vi "BRig_RT__Case_Exp__State_initTrial__LC_ENL__v4.vi"(6 "input_arrTrig":bool[](array[boolean]), 8 "input_dataTrial":u16[][](array[numeric]), 9 "input_dataExp":u16[](array[numeric]), 10 "input_dataLC":u16[](array[numeric]), 11 "input_dataCurrent":u16[](array[numeric])) -> (0 "output_dataTrial":u16[][](array[numeric]), 3 "output_dataCurrent":u16[](array[numeric]), 4 "output_arrTrig":bool[](array[boolean]))   [LabVIEW 2014]
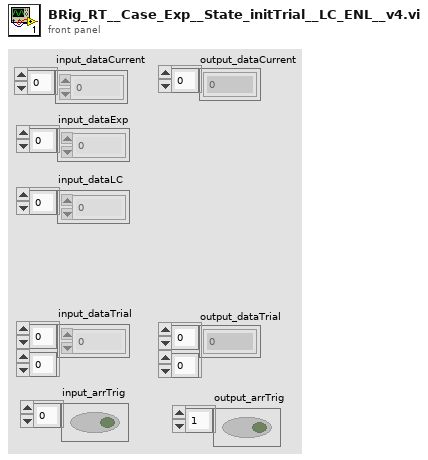
[diagram p1: front panel]
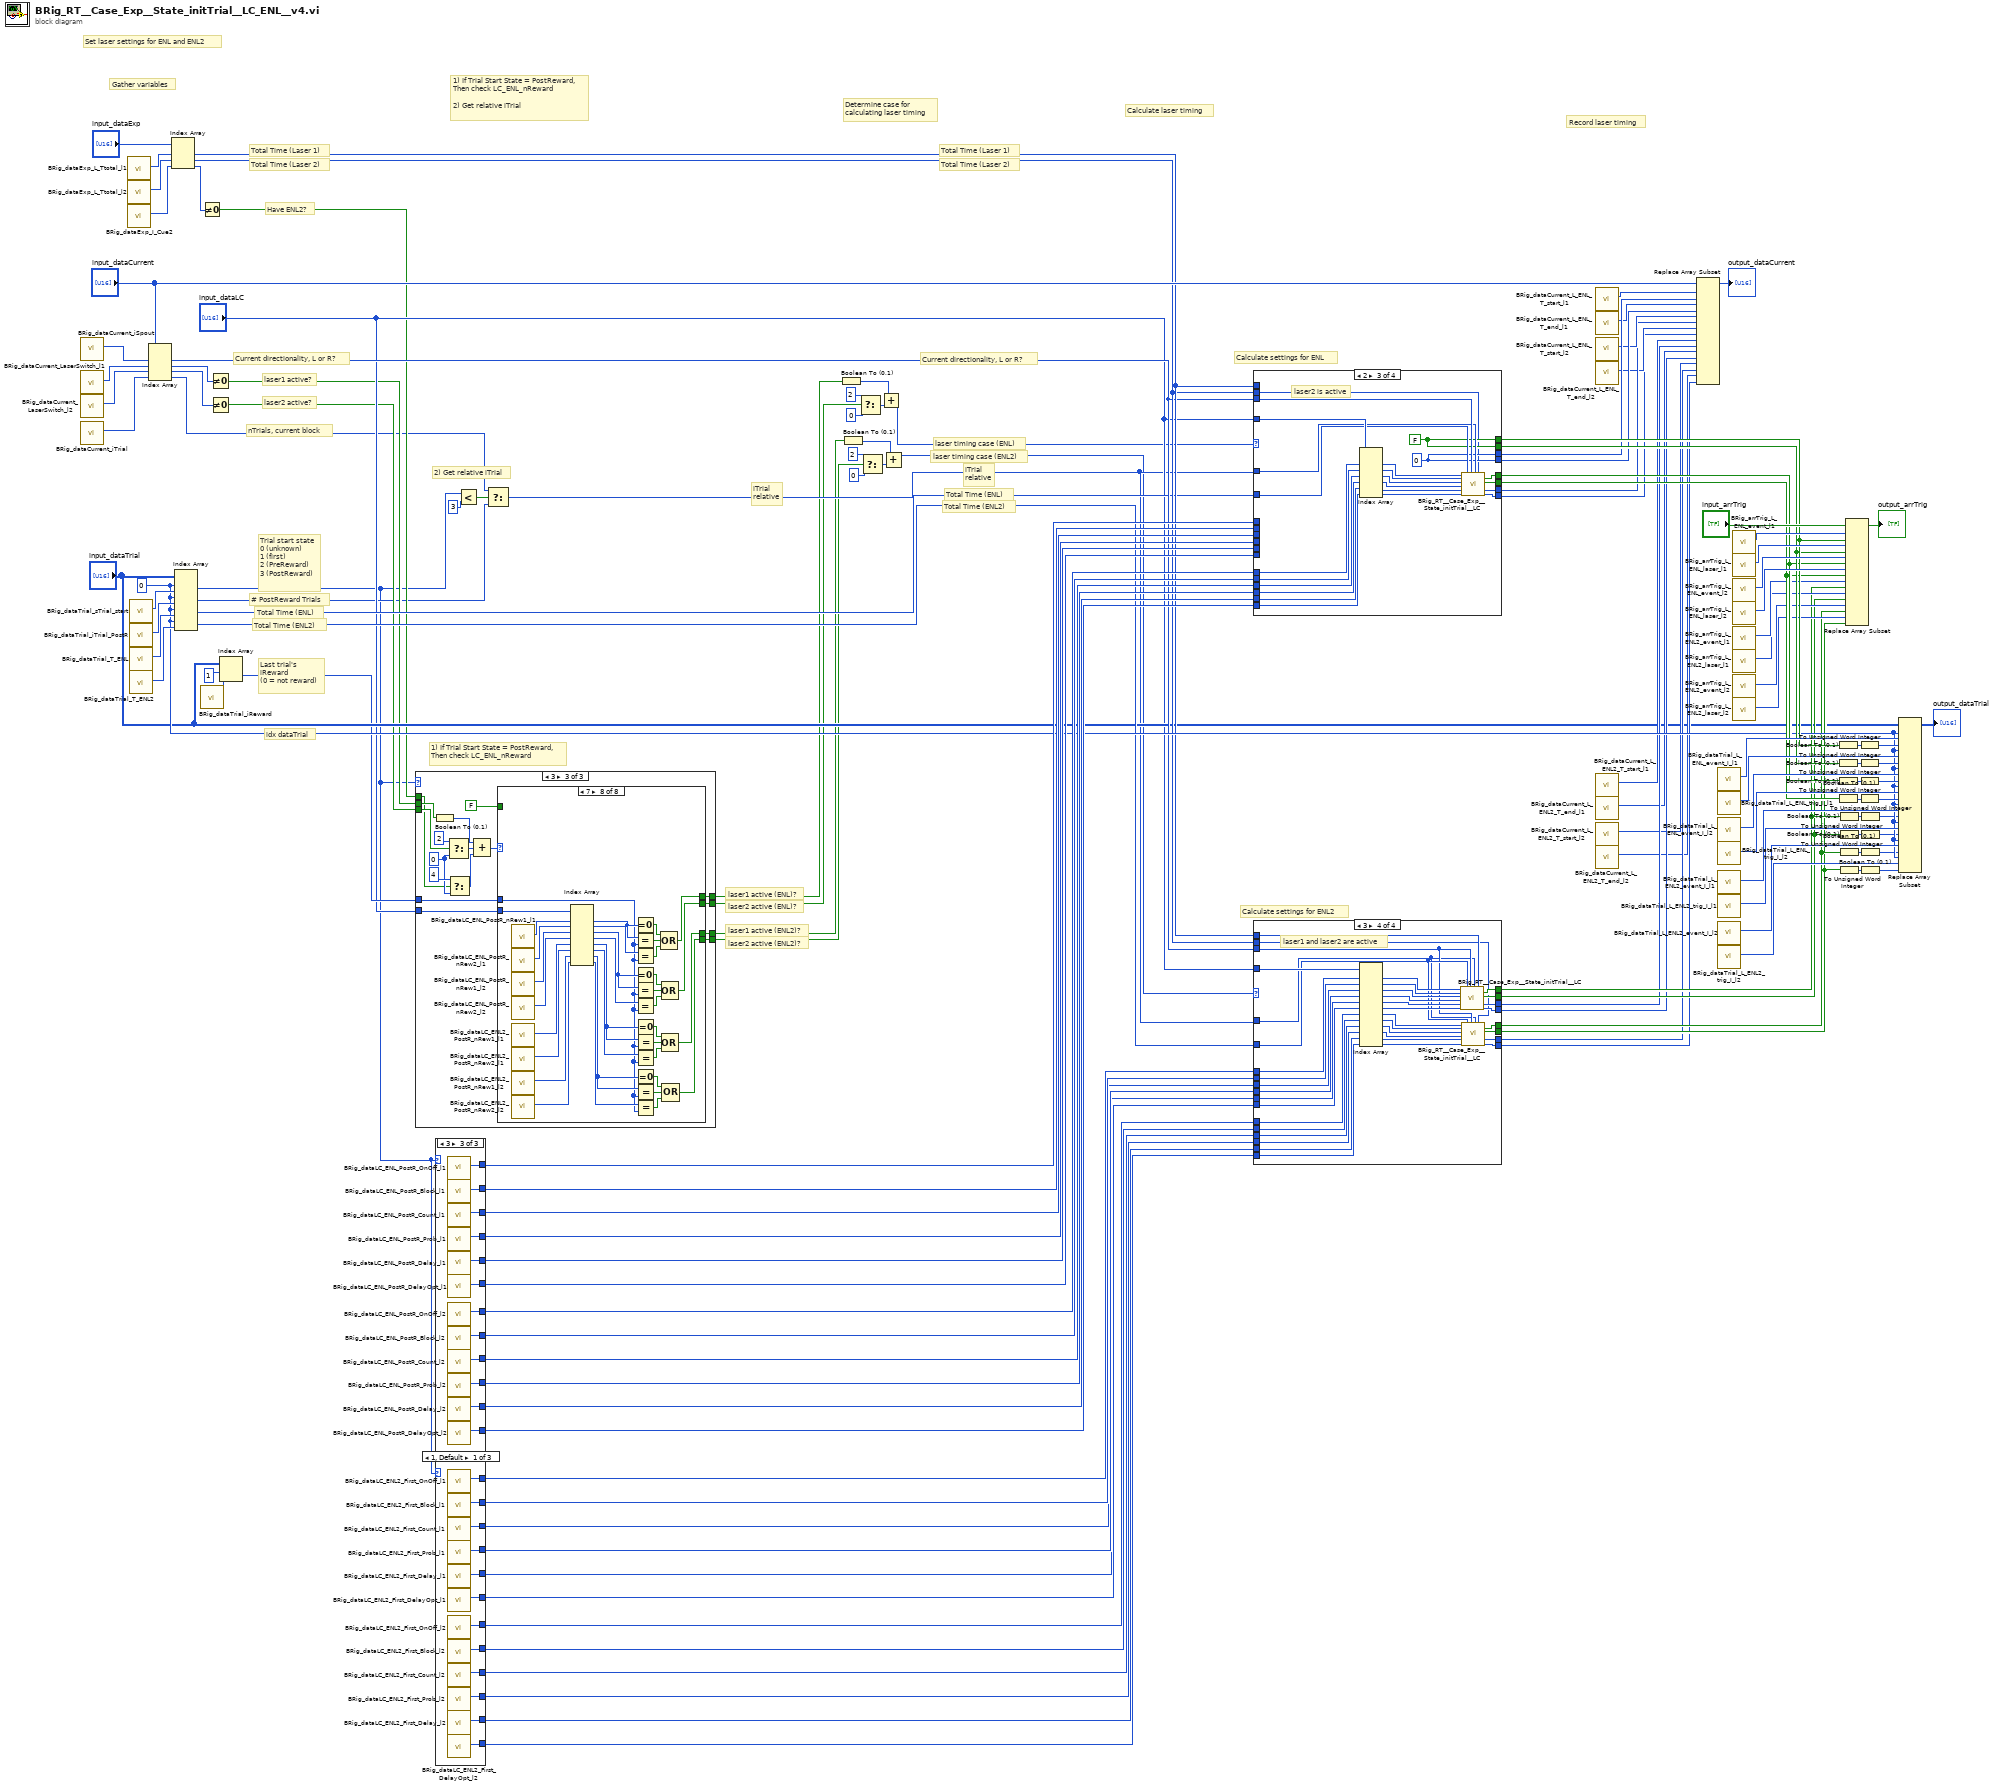
[diagram p0: block diagram]
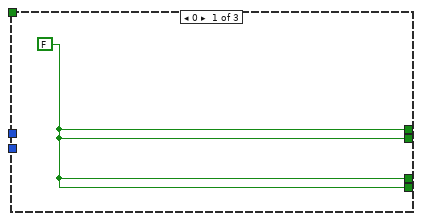
[diagram p2: hidden frame]
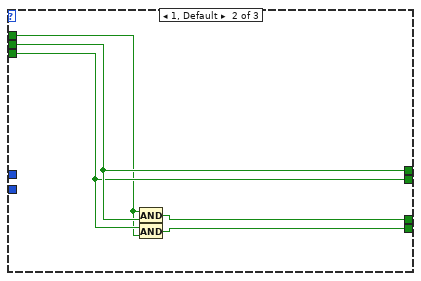
[diagram p3: hidden frame]
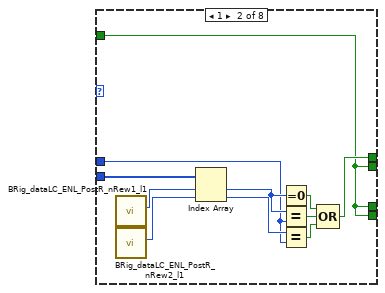
[diagram p5: hidden frame]
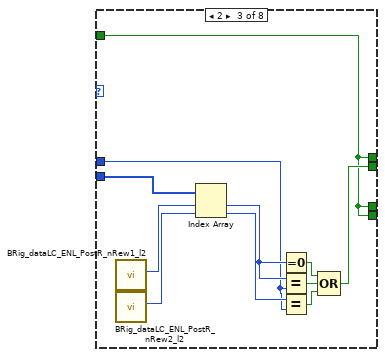
[diagram p6: hidden frame]
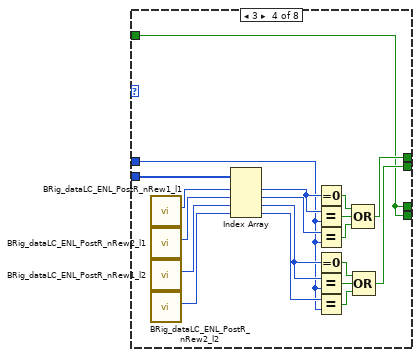
[diagram p7: hidden frame]
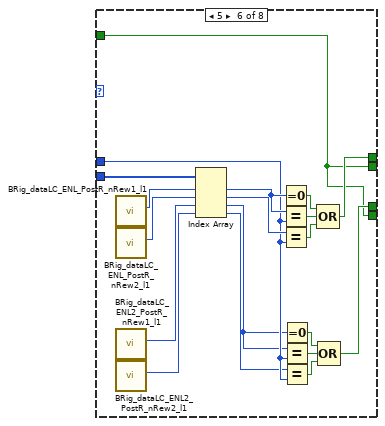
[diagram p9: hidden frame]
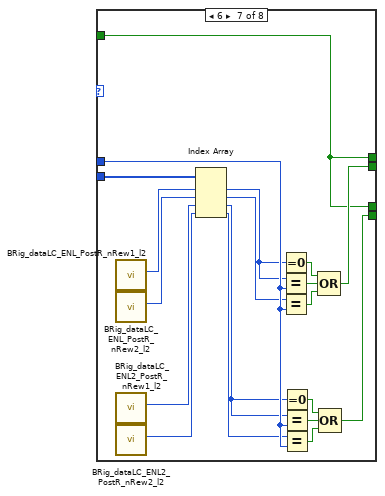
[diagram p10: hidden frame]
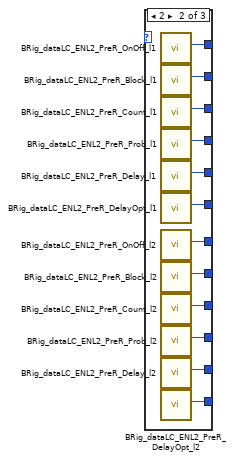
[diagram p11: hidden frame]
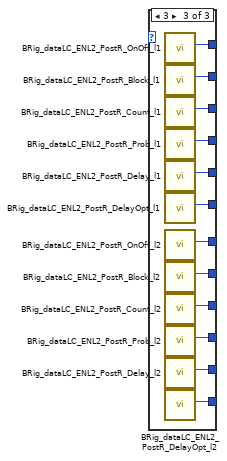
[diagram p12: hidden frame]
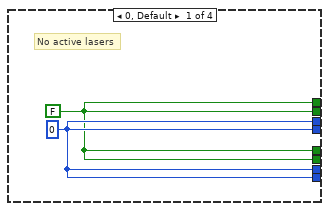
[diagram p13: hidden frame]
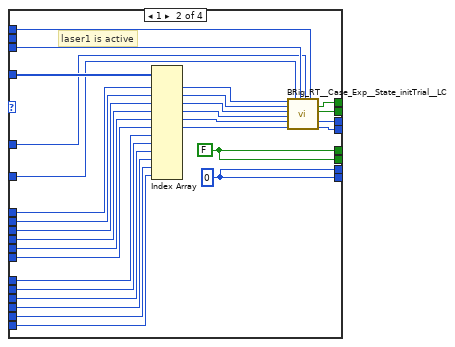
[diagram p14: hidden frame]
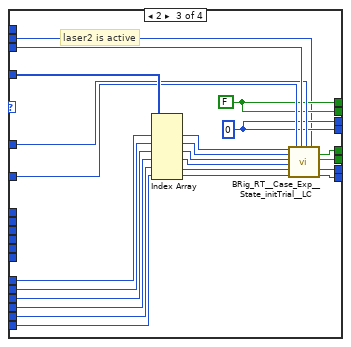
[diagram p15: hidden frame]
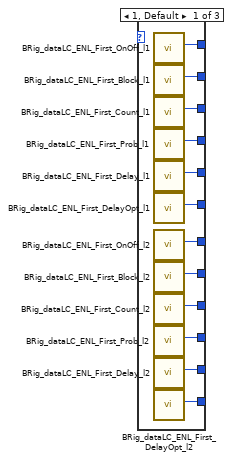
[diagram p16: hidden frame]
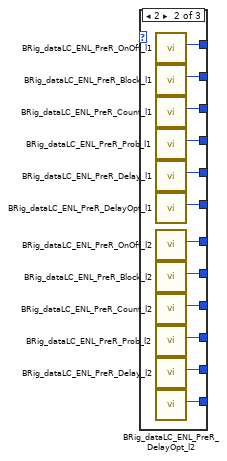
[diagram p17: hidden frame]
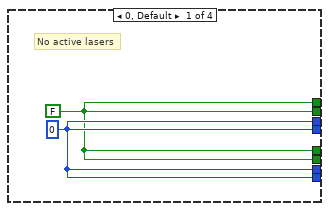
[diagram p18: hidden frame]
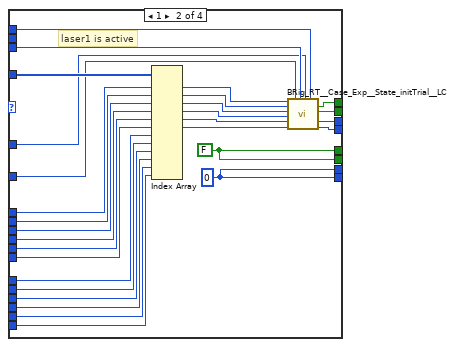
[diagram p19: hidden frame]
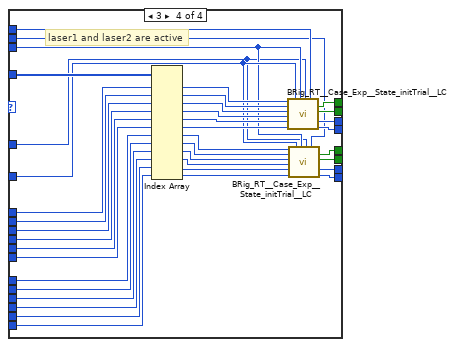
[diagram p20: hidden frame]
diagram:
  w61 = 0
  # "Record laser timing"
  # "Calculate laser timing"
  # "Total Time (ENL2)"
  # "Total Time (ENL)"
  # "iTrial\nrelative"
  # "Total Time (Laser 2)"
  # "Total Time (Laser 1)"
  # "Current directionality, L or R?"
  # "laser timing case (ENL2)"
  # "Determine case for\ncalculating laser timing"
  # "2) Get relative iTrial"
  # "1) If Trial Start State = PostReward,\nThen check LC_ENL_nReward"
  # "laser2 active (ENL2)?"
  # "laser1 active (ENL2)?"
  # "laser2 active (ENL)?"
  # "laser1 active (ENL)?"
  # "1) If Trial Start State = PostReward,\nThen check LC_ENL_nReward\n\n2) Get relative iTrial"
  # "Gather variables"
  # "Last trial's\niReward\n(0 = not reward)"
  # "nTrials, current block"
  # "idx dataTrial"
  # "Total Time (ENL2)"
  # "Total Time (ENL)"
  # "# PostReward Trials"
  # "Current directionality, L or R?"
  # "Have ENL2?"
  # "Total Time (Laser 2)"
  # "Total Time (Laser 1)"
  # "Calculate settings for ENL2"
  # "Calculate settings for ENL"
  # "Set laser settings for ENL and ENL2"
  # "iTrial\nrelative"
  # "laser timing case (ENL)"
  # "Trial start state\n0 (unknown)\n1 (first)\n2 (PreReward)\n3 (PostReward)"
  # "laser2 active?"
  # "laser1 active?"
  n1 = call "BRig_dataCurrent_iSpout.vi"() -> ("output_iSpout"=w125:i32)  [unwired: 11 in]
  n2 = call "BRig_dataCurrent_LaserSwitch_l1.vi"() -> ("output_LaserSwitch_l1"=w134:i32)  [unwired: 11 in]
  n3 = call "BRig_dataCurrent_LaserSwitch_l2.vi"() -> ("output_LaserSwitch_l2"=w133:i32)  [unwired: 11 in]
  n4 = call "BRig_dataCurrent_iTrial.vi"() -> ("output_iTrial"=w74:i32)  [unwired: 11 in]
  n5 = call "BRig_dataExp_L_Ttotal_l1.vi"() -> ("output_L_Ttotal_l1"=w78:i32)  [unwired: 11 in]
  n6 = call "BRig_dataExp_L_Ttotal_l2.vi"() -> ("output_L_Ttotal_l2"=w79:i32)  [unwired: 11 in]
  n7 = call "BRig_dataExp_I_Cue2.vi"() -> ("output_I_Cue2"=w28:i32)  [unwired: 11 in]
  n8 = call "BRig_dataTrial_sTrial_start.vi"() -> ("output_sTrial_start"=w130:i32)  [unwired: 11 in]
  n9 = call "BRig_dataTrial_iTrial_PostR.vi"() -> ("output_iTrial_PostR"=w75:i32)  [unwired: 11 in]
  n10 = call "BRig_dataTrial_T_ENL.vi"() -> ("output_T_ENL"=w76:i32)  [unwired: 11 in]
  n11 = call "BRig_dataTrial_T_ENL2.vi"() -> ("output_T_ENL2"=w73:i32)  [unwired: 11 in]
  n12 = Index Array(array="input_dataCurrent", index #1=w125, index #2=w134, index #3=w133, index #4=w74) -> (element #1=w53:u16, element #2=w132:u16, element #3=w131:u16, element #4=w14:u16)
  n13 = Index Array(array="input_dataExp", index #1=w78, index #2=w79, index #3=w28) -> (element #1=w55:u16, element #2=w54:u16, element #3=w27:u16)
  n14 = Index Array(array="input_dataTrial", index (row) #1=w61, index (col) #1=w130, index (row) #2=w61, index (col) #2=w75, index (row) #3=w61, index (col) #3=w76, index (row) #4=w61, index (col) #4=w73) -> (element #1=w12:u16, element #2=w13:u16, element #3=w26:u16, element #4=w25:u16)
  n15 = Not Equal To 0?(x=w27) -> (x != 0?=w17:bool)
  n16 = call "BRig_dataTrial_iReward.vi"() -> ("output_iReward"=w23:i32)  [unwired: 11 in]
  n17 = Not Equal To 0?(x=w132) -> (x != 0?=w18:bool)
  n18 = Not Equal To 0?(x=w131) -> (x != 0?=w19:bool)
  n19 = Index Array(array="input_dataTrial", index (row)=1 ("disabled index (row)"), index (col)=w23) -> (element=w21:u16)
  n20 = case shown="3" w12 {
    tunnel: w21 -> [_ _ w149]
    tunnel: "input_dataLC" -> [_ _ w150]
    tunnel: w19 -> [_ w139 w142]
    tunnel: w18 -> [_ w140 w143]
    tunnel: w17 -> [_ w138 w141]
    tunnel: [w135 w140 w148] -> w10
    tunnel: [w135 w139 w147] -> w9
    tunnel: [w135 w137 w146] -> w4
    tunnel: [w135 w136 w145] -> w3
    frame 0 {
      w135 = FALSE
    }
    frame 1, Default {
      n21 = And(x=w138, y=w140) -> (x .and. y?=w137:bool)
      n22 = And(x=w139, y=w138) -> (x .and. y?=w136:bool)
    }
    frame 3 {
      w155 = i16 0 ("f")
      n23 = Boolean To (0,1)(Boolean=w143) -> (0, 1=w153:i16)
      n24 = Select(t=i16 2, s=w142, f=w155) -> (s? t:f=w154:i16)
      n25 = Select(t=i16 4, s=w141, f=w155) -> (s? t:f=w152:i16)
      n26 = Compound Arithmetic op=ADD(w153, w154, w152) -> (w151:i16)
      n27 = case shown="7" w151 {
        tunnel: w150 -> [_ w162 w173 w185 _ w212 w235 w258]
        tunnel: w149 -> [_ w161 w172 w184 _ w208 w231 w243]
        tunnel: [w158 w160 w170 w183 w200 w207 w228 w242] -> w148
        tunnel: [w158 w159 w171 w182 w200 w205 w230 w241] -> w147
        tunnel: [w158 w159 w170 w181 w200 w206 w228 w240] -> w146
        tunnel: [w158 w159 w170 w181 w200 w205 w229 w239] -> w145
        tunnel: FALSE -> [w158 w159 w170 w181 w200 w205 w228 _]
        frame 0, Default {
        }
        frame 1 {
          n28 = call "BRig_dataLC_ENL_PostR_nRew1_l1.vi"() -> ("output_ENL_PostR_nRew1_l1"=w169:i32)  [unwired: 11 in]
          n29 = call "BRig_dataLC_ENL_PostR_nRew2_l1.vi"() -> ("output_ENL_PostR_nRew2_l1"=w168:i32)  [unwired: 11 in]
          n30 = Index Array(array=w162, index #1=w169, index #2=w168) -> (element #1=w164:u16, element #2=w163:u16)
          n31 = Equal To 0?(x=w164) -> (x = 0?=w165:bool)
          n32 = Equal?(x=w164, y=w161) -> (x = y?=w166:bool)
          n33 = Equal?(x=w163, y=w161) -> (x = y?=w167:bool)
          n34 = Compound Arithmetic op=OR(w165, w166, w167) -> (w160:bool)
        }
        frame 2 {
          n35 = call "BRig_dataLC_ENL_PostR_nRew1_l2.vi"() -> ("output_ENL_PostR_nRew1_l2"=w180:i32)  [unwired: 11 in]
          n36 = call "BRig_dataLC_ENL_PostR_nRew2_l2.vi"() -> ("output_ENL_PostR_nRew2_l2"=w179:i32)  [unwired: 11 in]
          n37 = Index Array(array=w173, index #1=w180, index #2=w179) -> (element #1=w174:u16, element #2=w175:u16)
          n38 = Equal To 0?(x=w174) -> (x = 0?=w177:bool)
          n39 = Equal?(x=w174, y=w172) -> (x = y?=w176:bool)
          n40 = Equal?(x=w175, y=w172) -> (x = y?=w178:bool)
          n41 = Compound Arithmetic op=OR(w177, w176, w178) -> (w171:bool)
        }
        frame 3 {
          n42 = call "BRig_dataLC_ENL_PostR_nRew1_l1.vi"() -> ("output_ENL_PostR_nRew1_l1"=w199:i32)  [unwired: 11 in]
          n43 = call "BRig_dataLC_ENL_PostR_nRew2_l1.vi"() -> ("output_ENL_PostR_nRew2_l1"=w198:i32)  [unwired: 11 in]
          n44 = call "BRig_dataLC_ENL_PostR_nRew1_l2.vi"() -> ("output_ENL_PostR_nRew1_l2"=w197:i32)  [unwired: 11 in]
          n45 = call "BRig_dataLC_ENL_PostR_nRew2_l2.vi"() -> ("output_ENL_PostR_nRew2_l2"=w196:i32)  [unwired: 11 in]
          n46 = Index Array(array=w185, index #1=w199, index #2=w198, index #3=w197, index #4=w196) -> (element #1=w189:u16, element #2=w188:u16, element #3=w186:u16, element #4=w187:u16)
          n47 = Equal To 0?(x=w189) -> (x = 0?=w190:bool)
          n48 = Equal?(x=w189, y=w184) -> (x = y?=w191:bool)
          n49 = Equal?(x=w188, y=w184) -> (x = y?=w192:bool)
          n50 = Equal To 0?(x=w186) -> (x = 0?=w194:bool)
          n51 = Equal?(x=w186, y=w184) -> (x = y?=w193:bool)
          n52 = Equal?(x=w187, y=w184) -> (x = y?=w195:bool)
          n53 = Compound Arithmetic op=OR(w190, w191, w192) -> (w183:bool)
          n54 = Compound Arithmetic op=OR(w194, w193, w195) -> (w182:bool)
        }
        frame 4 {
        }
        frame 5 {
          n55 = call "BRig_dataLC_ENL_PostR_nRew1_l1.vi"() -> ("output_ENL_PostR_nRew1_l1"=w219:i32)  [unwired: 11 in]
          n56 = call "BRig_dataLC_ENL_PostR_nRew2_l1.vi"() -> ("output_ENL_PostR_nRew2_l1"=w218:i32)  [unwired: 11 in]
          n57 = call "BRig_dataLC_ENL2_PostR_nRew1_l1.vi"() -> ("output_ENL2_PostR_nRew1_l1"=w204:i32)  [unwired: 11 in]
          n58 = call "BRig_dataLC_ENL2_PostR_nRew2_l1.vi"() -> ("output_ENL2_PostR_nRew2_l1"=w203:i32)  [unwired: 11 in]
          n59 = Index Array(array=w212, index #1=w219, index #2=w218, index #3=w204, index #4=w203) -> (element #1=w214:u16, element #2=w213:u16, element #3=w202:u16, element #4=w201:u16)
          n60 = Equal To 0?(x=w214) -> (x = 0?=w215:bool)
          n61 = Equal?(x=w214, y=w208) -> (x = y?=w216:bool)
          n62 = Equal?(x=w213, y=w208) -> (x = y?=w217:bool)
          n63 = Equal To 0?(x=w202) -> (x = 0?=w211:bool)
          n64 = Equal?(x=w202, y=w208) -> (x = y?=w210:bool)
          n65 = Equal?(x=w201, y=w208) -> (x = y?=w209:bool)
          n66 = Compound Arithmetic op=OR(w215, w216, w217) -> (w207:bool)
          n67 = Compound Arithmetic op=OR(w211, w210, w209) -> (w206:bool)
        }
        frame 6 {
          n68 = call "BRig_dataLC_ENL_PostR_nRew1_l2.vi"() -> ("output_ENL_PostR_nRew1_l2"=w227:i32)  [unwired: 11 in]
          n69 = call "BRig_dataLC_ENL_PostR_nRew2_l2.vi"() -> ("output_ENL_PostR_nRew2_l2"=w226:i32)  [unwired: 11 in]
          n70 = call "BRig_dataLC_ENL2_PostR_nRew1_l2.vi"() -> ("output_ENL2_PostR_nRew1_l2"=w223:i32)  [unwired: 11 in]
          n71 = call "BRig_dataLC_ENL2_PostR_nRew2_l2.vi"() -> ("output_ENL2_PostR_nRew2_l2"=w222:i32)  [unwired: 11 in]
          n72 = Index Array(array=w235, index #1=w227, index #2=w226, index #3=w223, index #4=w222) -> (element #1=w225:u16, element #2=w224:u16, element #3=w221:u16, element #4=w220:u16)
          n73 = Equal To 0?(x=w225) -> (x = 0?=w237:bool)
          n74 = Equal?(x=w225, y=w231) -> (x = y?=w236:bool)
          n75 = Equal?(x=w224, y=w231) -> (x = y?=w238:bool)
          n76 = Equal To 0?(x=w221) -> (x = 0?=w233:bool)
          n77 = Equal?(x=w221, y=w231) -> (x = y?=w234:bool)
          n78 = Equal?(x=w220, y=w231) -> (x = y?=w232:bool)
          n79 = Compound Arithmetic op=OR(w237, w236, w238) -> (w230:bool)
          n80 = Compound Arithmetic op=OR(w233, w234, w232) -> (w229:bool)
        }
        frame 7 {
          n81 = call "BRig_dataLC_ENL_PostR_nRew1_l1.vi"() -> ("output_ENL_PostR_nRew1_l1"=w272:i32)  [unwired: 11 in]
          n82 = call "BRig_dataLC_ENL_PostR_nRew2_l1.vi"() -> ("output_ENL_PostR_nRew2_l1"=w271:i32)  [unwired: 11 in]
          n83 = call "BRig_dataLC_ENL_PostR_nRew1_l2.vi"() -> ("output_ENL_PostR_nRew1_l2"=w270:i32)  [unwired: 11 in]
          n84 = call "BRig_dataLC_ENL_PostR_nRew2_l2.vi"() -> ("output_ENL_PostR_nRew2_l2"=w269:i32)  [unwired: 11 in]
          n85 = call "BRig_dataLC_ENL2_PostR_nRew1_l1.vi"() -> ("output_ENL2_PostR_nRew1_l1"=w257:i32)  [unwired: 11 in]
          n86 = call "BRig_dataLC_ENL2_PostR_nRew2_l1.vi"() -> ("output_ENL2_PostR_nRew2_l1"=w256:i32)  [unwired: 11 in]
          n87 = call "BRig_dataLC_ENL2_PostR_nRew1_l2.vi"() -> ("output_ENL2_PostR_nRew1_l2"=w255:i32)  [unwired: 11 in]
          n88 = call "BRig_dataLC_ENL2_PostR_nRew2_l2.vi"() -> ("output_ENL2_PostR_nRew2_l2"=w254:i32)  [unwired: 11 in]
          n89 = Index Array(array=w258, index #1=w272, index #2=w271, index #3=w270, index #4=w269, index #5=w257, index #6=w256, index #7=w255, index #8=w254) -> (element #1=w262:u16, element #2=w261:u16, element #3=w259:u16, element #4=w260:u16, element #5=w247:u16, element #6=w246:u16, element #7=w244:u16, element #8=w245:u16)
          n90 = Equal To 0?(x=w262) -> (x = 0?=w263:bool)
          n91 = Equal?(x=w262, y=w243) -> (x = y?=w264:bool)
          n92 = Equal?(x=w261, y=w243) -> (x = y?=w265:bool)
          n93 = Equal To 0?(x=w259) -> (x = 0?=w267:bool)
          n94 = Equal?(x=w259, y=w243) -> (x = y?=w266:bool)
          n95 = Equal?(x=w260, y=w243) -> (x = y?=w268:bool)
          n96 = Equal To 0?(x=w247) -> (x = 0?=w253:bool)
          n97 = Equal?(x=w247, y=w243) -> (x = y?=w252:bool)
          n98 = Equal?(x=w246, y=w243) -> (x = y?=w251:bool)
          n99 = Equal To 0?(x=w244) -> (x = 0?=w249:bool)
          n100 = Equal?(x=w244, y=w243) -> (x = y?=w250:bool)
          n101 = Equal?(x=w245, y=w243) -> (x = y?=w248:bool)
          n102 = Compound Arithmetic op=OR(w263, w264, w265) -> (w242:bool)
          n103 = Compound Arithmetic op=OR(w267, w266, w268) -> (w241:bool)
          n104 = Compound Arithmetic op=OR(w253, w252, w251) -> (w240:bool)
          n105 = Compound Arithmetic op=OR(w249, w250, w248) -> (w239:bool)
        }
      }
    }
  }
  n106 = case shown="3" w12 {
    tunnel: [w284 w296 w308] -> w91
    tunnel: [w283 w295 w297] -> w90
    tunnel: [w282 w294 w298] -> w89
    tunnel: [w281 w293 w299] -> w88
    tunnel: [w280 w292 w300] -> w87
    tunnel: [w279 w291 w301] -> w86
    tunnel: [w278 w290 w307] -> w85
    tunnel: [w277 w289 w306] -> w84
    tunnel: [w276 w288 w305] -> w83
    tunnel: [w275 w287 w304] -> w82
    tunnel: [w274 w286 w303] -> w81
    tunnel: [w273 w285 w302] -> w80
    frame 1, Default {
      n107 = call "BRig_dataLC_ENL_First_OnOff_l1.vi"() -> ("output_ENL_First_OnOff"=w284:i32)  [unwired: 11 in]
      n108 = call "BRig_dataLC_ENL_First_Block_l1.vi"() -> ("output_ENL_First_Block"=w283:i32)  [unwired: 11 in]
      n109 = call "BRig_dataLC_ENL_First_Count_l1.vi"() -> ("output_ENL_First_Count"=w282:i32)  [unwired: 11 in]
      n110 = call "BRig_dataLC_ENL_First_Prob_l1.vi"() -> ("output_ENL_First_Prob"=w281:i32)  [unwired: 11 in]
      n111 = call "BRig_dataLC_ENL_First_Delay_l1.vi"() -> ("output_ENL_First_Delay"=w280:i32)  [unwired: 11 in]
      n112 = call "BRig_dataLC_ENL_First_DelayOpt_l1.vi"() -> ("output_ENL_First_DelayOpt"=w279:i32)  [unwired: 11 in]
      n113 = call "BRig_dataLC_ENL_First_OnOff_l2.vi"() -> ("output_ENL_First_OnOff_l2"=w278:i32)  [unwired: 11 in]
      n114 = call "BRig_dataLC_ENL_First_Block_l2.vi"() -> ("output_ENL_First_Block_l2"=w277:i32)  [unwired: 11 in]
      n115 = call "BRig_dataLC_ENL_First_Count_l2.vi"() -> ("output_ENL_First_Count_l2"=w276:i32)  [unwired: 11 in]
      n116 = call "BRig_dataLC_ENL_First_Prob_l2.vi"() -> ("output_ENL_First_Prob_l2"=w275:i32)  [unwired: 11 in]
      n117 = call "BRig_dataLC_ENL_First_Delay_l2.vi"() -> ("output_ENL_First_Delay_l2"=w274:i32)  [unwired: 11 in]
      n118 = call "BRig_dataLC_ENL_First_DelayOpt_l2.vi"() -> ("output_ENL_First_DelayOpt_l2"=w273:i32)  [unwired: 11 in]
    }
    frame 2 {
      n119 = call "BRig_dataLC_ENL_PreR_OnOff_l1.vi"() -> ("output_ENL_PreR_OnOff"=w296:i32)  [unwired: 11 in]
      n120 = call "BRig_dataLC_ENL_PreR_Block_l1.vi"() -> ("output_ENL_PreR_Block"=w295:i32)  [unwired: 11 in]
      n121 = call "BRig_dataLC_ENL_PreR_Count_l1.vi"() -> ("output_ENL_PreR_Count"=w294:i32)  [unwired: 11 in]
      n122 = call "BRig_dataLC_ENL_PreR_Prob_l1.vi"() -> ("output_ENL_PreR_Prob"=w293:i32)  [unwired: 11 in]
      n123 = call "BRig_dataLC_ENL_PreR_Delay_l1.vi"() -> ("output_ENL_PreR_Delay"=w292:i32)  [unwired: 11 in]
      n124 = call "BRig_dataLC_ENL_PreR_DelayOpt_l1.vi"() -> ("output_ENL_PreR_DelayOpt"=w291:i32)  [unwired: 11 in]
      n125 = call "BRig_dataLC_ENL_PreR_OnOff_l2.vi"() -> ("output_ENL_PreR_OnOff_l2"=w290:i32)  [unwired: 11 in]
      n126 = call "BRig_dataLC_ENL_PreR_Block_l2.vi"() -> ("output_ENL_PreR_Block_l2"=w289:i32)  [unwired: 11 in]
      n127 = call "BRig_dataLC_ENL_PreR_Count_l2.vi"() -> ("output_ENL_PreR_Count_l2"=w288:i32)  [unwired: 11 in]
      n128 = call "BRig_dataLC_ENL_PreR_Prob_l2.vi"() -> ("output_ENL_PreR_Prob_l2"=w287:i32)  [unwired: 11 in]
      n129 = call "BRig_dataLC_ENL_PreR_Delay_l2.vi"() -> ("output_ENL_PreR_Delay_l2"=w286:i32)  [unwired: 11 in]
      n130 = call "BRig_dataLC_ENL_PreR_DelayOpt_l2.vi"() -> ("output_ENL_PreR_DelayOpt_l2"=w285:i32)  [unwired: 11 in]
    }
    frame 3 {
      n131 = call "BRig_dataLC_ENL_PostR_OnOff_l1.vi"() -> ("output_ENL_PostR_OnOff"=w308:i32)  [unwired: 11 in]
      n132 = call "BRig_dataLC_ENL_PostR_Block_l1.vi"() -> ("output_ENL_PostR_Block"=w297:i32)  [unwired: 11 in]
      n133 = call "BRig_dataLC_ENL_PostR_Count_l1.vi"() -> ("output_ENL_PostR_Count"=w298:i32)  [unwired: 11 in]
      n134 = call "BRig_dataLC_ENL_PostR_Prob_l1.vi"() -> ("output_ENL_PostR_Prob"=w299:i32)  [unwired: 11 in]
      n135 = call "BRig_dataLC_ENL_PostR_Delay_l1.vi"() -> ("output_ENL_PostR_Delay"=w300:i32)  [unwired: 11 in]
      n136 = call "BRig_dataLC_ENL_PostR_DelayOpt_l1.vi"() -> ("output_ENL_PostR_DelayOpt"=w301:i32)  [unwired: 11 in]
      n137 = call "BRig_dataLC_ENL_PostR_OnOff_l2.vi"() -> ("output_ENL_PostR_OnOff_l2"=w307:i32)  [unwired: 11 in]
      n138 = call "BRig_dataLC_ENL_PostR_Block_l2.vi"() -> ("output_ENL_PostR_Block_l2"=w306:i32)  [unwired: 11 in]
      n139 = call "BRig_dataLC_ENL_PostR_Count_l2.vi"() -> ("output_ENL_PostR_Count_l2"=w305:i32)  [unwired: 11 in]
      n140 = call "BRig_dataLC_ENL_PostR_Prob_l2.vi"() -> ("output_ENL_PostR_Prob_l2"=w304:i32)  [unwired: 11 in]
      n141 = call "BRig_dataLC_ENL_PostR_Delay_l2.vi"() -> ("output_ENL_PostR_Delay_l2"=w303:i32)  [unwired: 11 in]
      n142 = call "BRig_dataLC_ENL_PostR_DelayOpt_l2.vi"() -> ("output_ENL_PostR_DelayOpt_l2"=w302:i32)  [unwired: 11 in]
    }
  }
  n143 = case shown="1, Default" w12 {
    tunnel: [w320 w332 w344] -> w52
    tunnel: [w319 w331 w343] -> w51
    tunnel: [w318 w330 w342] -> w50
    tunnel: [w317 w329 w341] -> w49
    tunnel: [w316 w328 w340] -> w48
    tunnel: [w315 w327 w339] -> w47
    tunnel: [w314 w326 w338] -> w46
    tunnel: [w313 w325 w337] -> w45
    tunnel: [w312 w324 w336] -> w44
    tunnel: [w311 w323 w335] -> w43
    tunnel: [w310 w322 w334] -> w42
    tunnel: [w309 w321 w333] -> w41
    frame 1, Default {
      n144 = call "BRig_dataLC_ENL2_First_OnOff_l1.vi"() -> ("output_ENL2_First_OnOff"=w320:i32)  [unwired: 11 in]
      n145 = call "BRig_dataLC_ENL2_First_Block_l1.vi"() -> ("output_ENL2_First_Block"=w319:i32)  [unwired: 11 in]
      n146 = call "BRig_dataLC_ENL2_First_Count_l1.vi"() -> ("output_ENL2_First_Count"=w318:i32)  [unwired: 11 in]
      n147 = call "BRig_dataLC_ENL2_First_Prob_l1.vi"() -> ("output_ENL2_First_Prob"=w317:i32)  [unwired: 11 in]
      n148 = call "BRig_dataLC_ENL2_First_Delay_l1.vi"() -> ("output_ENL2_First_Delay"=w316:i32)  [unwired: 11 in]
      n149 = call "BRig_dataLC_ENL2_First_DelayOpt_l1.vi"() -> ("output_ENL2_First_DelayOpt"=w315:i32)  [unwired: 11 in]
      n150 = call "BRig_dataLC_ENL2_First_OnOff_l2.vi"() -> ("output_ENL2_First_OnOff_l2"=w314:i32)  [unwired: 11 in]
      n151 = call "BRig_dataLC_ENL2_First_Block_l2.vi"() -> ("output_ENL2_First_Block_l2"=w313:i32)  [unwired: 11 in]
      n152 = call "BRig_dataLC_ENL2_First_Count_l2.vi"() -> ("output_ENL2_First_Count_l2"=w312:i32)  [unwired: 11 in]
      n153 = call "BRig_dataLC_ENL2_First_Prob_l2.vi"() -> ("output_ENL2_First_Prob_l2"=w311:i32)  [unwired: 11 in]
      n154 = call "BRig_dataLC_ENL2_First_Delay_l2.vi"() -> ("output_ENL2_First_Delay_l2"=w310:i32)  [unwired: 11 in]
      n155 = call "BRig_dataLC_ENL2_First_DelayOpt_l2.vi"() -> ("output_ENL2_First_DelayOpt_l2"=w309:i32)  [unwired: 11 in]
    }
    frame 2 {
      n156 = call "BRig_dataLC_ENL2_PreR_OnOff_l1.vi"() -> ("output_ENL2_PreR_OnOff"=w332:i32)  [unwired: 11 in]
      n157 = call "BRig_dataLC_ENL2_PreR_Block_l1.vi"() -> ("output_ENL2_PreR_Block"=w331:i32)  [unwired: 11 in]
      n158 = call "BRig_dataLC_ENL2_PreR_Count_l1.vi"() -> ("output_ENL2_PreR_Count"=w330:i32)  [unwired: 11 in]
      n159 = call "BRig_dataLC_ENL2_PreR_Prob_l1.vi"() -> ("output_ENL2_PreR_Prob"=w329:i32)  [unwired: 11 in]
      n160 = call "BRig_dataLC_ENL2_PreR_Delay_l1.vi"() -> ("output_ENL2_PreR_Delay"=w328:i32)  [unwired: 11 in]
      n161 = call "BRig_dataLC_ENL2_PreR_DelayOpt_l1.vi"() -> ("output_ENL2_PreR_DelayOpt"=w327:i32)  [unwired: 11 in]
      n162 = call "BRig_dataLC_ENL2_PreR_OnOff_l2.vi"() -> ("output_ENL2_PreR_OnOff_l2"=w326:i32)  [unwired: 11 in]
      n163 = call "BRig_dataLC_ENL2_PreR_Block_l2.vi"() -> ("output_ENL2_PreR_Block_l2"=w325:i32)  [unwired: 11 in]
      n164 = call "BRig_dataLC_ENL2_PreR_Count_l2.vi"() -> ("output_ENL2_PreR_Count_l2"=w324:i32)  [unwired: 11 in]
      n165 = call "BRig_dataLC_ENL2_PreR_Prob_l2.vi"() -> ("output_ENL2_PreR_Prob_l2"=w323:i32)  [unwired: 11 in]
      n166 = call "BRig_dataLC_ENL2_PreR_Delay_l2.vi"() -> ("output_ENL2_PreR_Delay_l2"=w322:i32)  [unwired: 11 in]
      n167 = call "BRig_dataLC_ENL2_PreR_DelayOpt_l2.vi"() -> ("output_ENL2_PreR_DelayOpt_l2"=w321:i32)  [unwired: 11 in]
    }
    frame 3 {
      n168 = call "BRig_dataLC_ENL2_PostR_OnOff_l1.vi"() -> ("output_ENL2_PostR_OnOff"=w344:i32)  [unwired: 11 in]
      n169 = call "BRig_dataLC_ENL2_PostR_Block_l1.vi"() -> ("output_ENL2_PostR_Block"=w343:i32)  [unwired: 11 in]
      n170 = call "BRig_dataLC_ENL2_PostR_Count_l1.vi"() -> ("output_ENL2_PostR_Count"=w342:i32)  [unwired: 11 in]
      n171 = call "BRig_dataLC_ENL2_PostR_Prob_l1.vi"() -> ("output_ENL2_PostR_Prob"=w341:i32)  [unwired: 11 in]
      n172 = call "BRig_dataLC_ENL2_PostR_Delay_l1.vi"() -> ("output_ENL2_PostR_Delay"=w340:i32)  [unwired: 11 in]
      n173 = call "BRig_dataLC_ENL2_PostR_DelayOpt_l1.vi"() -> ("output_ENL2_PostR_DelayOpt"=w339:i32)  [unwired: 11 in]
      n174 = call "BRig_dataLC_ENL2_PostR_OnOff_l2.vi"() -> ("output_ENL2_PostR_OnOff_l2"=w338:i32)  [unwired: 11 in]
      n175 = call "BRig_dataLC_ENL2_PostR_Block_l2.vi"() -> ("output_ENL2_PostR_Block_l2"=w337:i32)  [unwired: 11 in]
      n176 = call "BRig_dataLC_ENL2_PostR_Count_l2.vi"() -> ("output_ENL2_PostR_Count_l2"=w336:i32)  [unwired: 11 in]
      n177 = call "BRig_dataLC_ENL2_PostR_Prob_l2.vi"() -> ("output_ENL2_PostR_Prob_l2"=w335:i32)  [unwired: 11 in]
      n178 = call "BRig_dataLC_ENL2_PostR_Delay_l2.vi"() -> ("output_ENL2_PostR_Delay_l2"=w334:i32)  [unwired: 11 in]
      n179 = call "BRig_dataLC_ENL2_PostR_DelayOpt_l2.vi"() -> ("output_ENL2_PostR_DelayOpt_l2"=w333:i32)  [unwired: 11 in]
    }
  }
  n180 = Less?(x=w12, y=u16 3) -> (x < y?=w15:bool)
  n181 = Select(t=w14, s=w15, f=w13) -> (s? t:f=w11:u16)
  n182 = Boolean To (0,1)(Boolean=w10) -> (0, 1=w127:i16)
  n183 = Boolean To (0,1)(Boolean=w4) -> (0, 1=w7:i16)
  n184 = Select(t=i16 2, s=w9, f=i16 0) -> (s? t:f=w128:i16)
  n185 = Select(t=i16 2, s=w3, f=i16 0) -> (s? t:f=w6:i16)
  n186 = Add(x=w127, y=w128) -> (x+y=w2:i16)
  n187 = Add(x=w7, y=w6) -> (x+y=w1:i16)
  n188 = case shown="2" w2 {
    tunnel: "input_dataLC" -> [_ w375 w398 w436]
    tunnel: w53 -> [_ w367 w390 w422]
    tunnel: w26 -> [_ w368 w391 w423]
    tunnel: w11 -> [_ w366 w389 w421]
    tunnel: [w345 w365 w378 w420] -> w113
    tunnel: [w345 w364 w378 w419] -> w107
    tunnel: [w346 w363 w377 w418] -> w98
    tunnel: [w346 w362 w377 w417] -> w96
    tunnel: [w345 w349 w388 w416] -> w103
    tunnel: [w346 w348 w387 w415] -> w94
    tunnel: [w345 w349 w386 w414] -> w105
    tunnel: [w346 w348 w385 w413] -> w92
    tunnel: w91 -> [_ w361 _ w412]
    tunnel: w90 -> [_ w360 _ w411]
    tunnel: w89 -> [_ w359 _ w410]
    tunnel: w88 -> [_ w358 _ w409]
    tunnel: w87 -> [_ w357 _ w408]
    tunnel: w86 -> [_ w356 _ w407]
    tunnel: w85 -> [_ w355 w384 w406]
    tunnel: w84 -> [_ w354 w383 w405]
    tunnel: w83 -> [_ w353 w382 w404]
    tunnel: w82 -> [_ w352 w381 w403]
    tunnel: w81 -> [_ w351 w380 w402]
    tunnel: w80 -> [_ w350 w379 w401]
    tunnel: w55 -> [_ w347 _ w400]
    tunnel: w54 -> [_ _ w376 w399]
    frame 0, Default {
      w346 = u16 0
      w345 = FALSE
      # "No active lasers"
    }
    frame 1 {
      w348 = u16 0
      w349 = FALSE
      # "laser1 is active"
      n189 = Index Array(array=w375, index #1=w361, index #2=w360, index #3=w359, index #4=w358, index #5=w357, index #6=w356, index #7=w355, index #8=w354, index #9=w353, index #10=w352, index #11=w351, index #12=w350) -> (element #1=w374:u16, element #2=w373:u16, element #3=w372:u16, element #4=w371:u16, element #5=w370:u16, element #6=w369:u16)  [unwired: 6 out]
      n190 = call "BRig_RT__Case_Exp__State_initTrial__LC.vi"("input_L_OnOff"=w374, "input_L_Block"=w373, "input_L_Count"=w372, "input_L_Prob"=w371, "input_L_Tdelay"=w370, "input_L_delayOpt"=w369, "input_T_state"=w368, "input_iSpout"=w367, "input_iTrial_relative"=w366, "input_L_T"=w347) -> ("output_LC_Event"=w365:bool, "output_LC_Laser"=w364:bool, "output_L_Tstart"=w363:u16, "output_L_Tend"=w362:u16)  [unwired: 6 in]
    }
    frame 2 {
      w377 = u16 0
      w378 = FALSE
      # "laser2 is active"
      n191 = Index Array(array=w398, index #1=w384, index #2=w383, index #3=w382, index #4=w381, index #5=w380, index #6=w379) -> (element #1=w392:u16, element #2=w393:u16, element #3=w394:u16, element #4=w395:u16, element #5=w396:u16, element #6=w397:u16)
      n192 = call "BRig_RT__Case_Exp__State_initTrial__LC.vi"("input_L_OnOff"=w392, "input_L_Block"=w393, "input_L_Count"=w394, "input_L_Prob"=w395, "input_L_Tdelay"=w396, "input_L_delayOpt"=w397, "input_T_state"=w391, "input_iSpout"=w390, "input_iTrial_relative"=w389, "input_L_T"=w376) -> ("output_LC_Event"=w386:bool, "output_LC_Laser"=w388:bool, "output_L_Tstart"=w387:u16, "output_L_Tend"=w385:u16)  [unwired: 6 in]
    }
    frame 3 {
      # "laser1 and laser2 are active"
      n193 = Index Array(array=w436, index #1=w412, index #2=w411, index #3=w410, index #4=w409, index #5=w408, index #6=w407, index #7=w406, index #8=w405, index #9=w404, index #10=w403, index #11=w402, index #12=w401) -> (element #1=w435:u16, element #2=w434:u16, element #3=w433:u16, element #4=w432:u16, element #5=w431:u16, element #6=w430:u16, element #7=w424:u16, element #8=w425:u16, element #9=w426:u16, element #10=w427:u16, element #11=w428:u16, element #12=w429:u16)
      n194 = call "BRig_RT__Case_Exp__State_initTrial__LC.vi"("input_L_OnOff"=w435, "input_L_Block"=w434, "input_L_Count"=w433, "input_L_Prob"=w432, "input_L_Tdelay"=w431, "input_L_delayOpt"=w430, "input_T_state"=w423, "input_iSpout"=w422, "input_iTrial_relative"=w421, "input_L_T"=w400) -> ("output_LC_Event"=w420:bool, "output_LC_Laser"=w419:bool, "output_L_Tstart"=w418:u16, "output_L_Tend"=w417:u16)  [unwired: 6 in]
      n195 = call "BRig_RT__Case_Exp__State_initTrial__LC.vi"("input_L_OnOff"=w424, "input_L_Block"=w425, "input_L_Count"=w426, "input_L_Prob"=w427, "input_L_Tdelay"=w428, "input_L_delayOpt"=w429, "input_T_state"=w423, "input_iSpout"=w422, "input_iTrial_relative"=w421, "input_L_T"=w399) -> ("output_LC_Event"=w414:bool, "output_LC_Laser"=w416:bool, "output_L_Tstart"=w415:u16, "output_L_Tend"=w413:u16)  [unwired: 6 in]
    }
  }
  n196 = case shown="3" w1 {
    tunnel: "input_dataLC" -> [_ w467 w490 w528]
    tunnel: w53 -> [_ w459 w482 w514]
    tunnel: w25 -> [_ w460 w483 w515]
    tunnel: w11 -> [_ w458 w481 w513]
    tunnel: [w437 w457 w470 w512] -> w40
    tunnel: [w437 w456 w470 w511] -> w39
    tunnel: [w438 w455 w469 w510] -> w35
    tunnel: [w438 w454 w469 w509] -> w33
    tunnel: [w437 w441 w480 w508] -> w37
    tunnel: [w438 w440 w479 w507] -> w31
    tunnel: [w437 w441 w478 w506] -> w38
    tunnel: [w438 w440 w477 w505] -> w29
    tunnel: w52 -> [_ w453 _ w504]
    tunnel: w51 -> [_ w452 _ w503]
    tunnel: w50 -> [_ w451 _ w502]
    tunnel: w49 -> [_ w450 _ w501]
    tunnel: w48 -> [_ w449 _ w500]
    tunnel: w47 -> [_ w448 _ w499]
    tunnel: w46 -> [_ w447 w476 w498]
    tunnel: w45 -> [_ w446 w475 w497]
    tunnel: w44 -> [_ w445 w474 w496]
    tunnel: w43 -> [_ w444 w473 w495]
    tunnel: w42 -> [_ w443 w472 w494]
    tunnel: w41 -> [_ w442 w471 w493]
    tunnel: w55 -> [_ w439 _ w492]
    tunnel: w54 -> [_ _ w468 w491]
    frame 0, Default {
      w438 = u16 0
      w437 = FALSE
      # "No active lasers"
    }
    frame 1 {
      w440 = u16 0
      w441 = FALSE
      # "laser1 is active"
      n197 = Index Array(array=w467, index #1=w453, index #2=w452, index #3=w451, index #4=w450, index #5=w449, index #6=w448, index #7=w447, index #8=w446, index #9=w445, index #10=w444, index #11=w443, index #12=w442) -> (element #1=w466:u16, element #2=w465:u16, element #3=w464:u16, element #4=w463:u16, element #5=w462:u16, element #6=w461:u16)  [unwired: 6 out]
      n198 = call "BRig_RT__Case_Exp__State_initTrial__LC.vi"("input_L_OnOff"=w466, "input_L_Block"=w465, "input_L_Count"=w464, "input_L_Prob"=w463, "input_L_Tdelay"=w462, "input_L_delayOpt"=w461, "input_T_state"=w460, "input_iSpout"=w459, "input_iTrial_relative"=w458, "input_L_T"=w439) -> ("output_LC_Event"=w457:bool, "output_LC_Laser"=w456:bool, "output_L_Tstart"=w455:u16, "output_L_Tend"=w454:u16)  [unwired: 6 in]
    }
    frame 2 {
      w469 = u16 0
      w470 = FALSE
      # "laser2 is active"
      n199 = Index Array(array=w490, index #1=w476, index #2=w475, index #3=w474, index #4=w473, index #5=w472, index #6=w471) -> (element #1=w484:u16, element #2=w485:u16, element #3=w486:u16, element #4=w487:u16, element #5=w488:u16, element #6=w489:u16)
      n200 = call "BRig_RT__Case_Exp__State_initTrial__LC.vi"("input_L_OnOff"=w484, "input_L_Block"=w485, "input_L_Count"=w486, "input_L_Prob"=w487, "input_L_Tdelay"=w488, "input_L_delayOpt"=w489, "input_T_state"=w483, "input_iSpout"=w482, "input_iTrial_relative"=w481, "input_L_T"=w468) -> ("output_LC_Event"=w478:bool, "output_LC_Laser"=w480:bool, "output_L_Tstart"=w479:u16, "output_L_Tend"=w477:u16)  [unwired: 6 in]
    }
    frame 3 {
      # "laser1 and laser2 are active"
      n201 = Index Array(array=w528, index #1=w504, index #2=w503, index #3=w502, index #4=w501, index #5=w500, index #6=w499, index #7=w498, index #8=w497, index #9=w496, index #10=w495, index #11=w494, index #12=w493) -> (element #1=w527:u16, element #2=w526:u16, element #3=w525:u16, element #4=w524:u16, element #5=w523:u16, element #6=w522:u16, element #7=w516:u16, element #8=w517:u16, element #9=w518:u16, element #10=w519:u16, element #11=w520:u16, element #12=w521:u16)
      n202 = call "BRig_RT__Case_Exp__State_initTrial__LC.vi"("input_L_OnOff"=w527, "input_L_Block"=w526, "input_L_Count"=w525, "input_L_Prob"=w524, "input_L_Tdelay"=w523, "input_L_delayOpt"=w522, "input_T_state"=w515, "input_iSpout"=w514, "input_iTrial_relative"=w513, "input_L_T"=w492) -> ("output_LC_Event"=w512:bool, "output_LC_Laser"=w511:bool, "output_L_Tstart"=w510:u16, "output_L_Tend"=w509:u16)  [unwired: 6 in]
      n203 = call "BRig_RT__Case_Exp__State_initTrial__LC.vi"("input_L_OnOff"=w516, "input_L_Block"=w517, "input_L_Count"=w518, "input_L_Prob"=w519, "input_L_Tdelay"=w520, "input_L_delayOpt"=w521, "input_T_state"=w515, "input_iSpout"=w514, "input_iTrial_relative"=w513, "input_L_T"=w491) -> ("output_LC_Event"=w506:bool, "output_LC_Laser"=w508:bool, "output_L_Tstart"=w507:u16, "output_L_Tend"=w505:u16)  [unwired: 6 in]
    }
  }
  n204 = call "BRig_dataCurrent_L_ENL_T_start_l1.vi"() -> ("output_L_ENL_T_start_l1"=w99:i32)  [unwired: 11 in]
  n205 = call "BRig_dataCurrent_L_ENL_T_end_l1.vi"() -> ("output_L_ENL_T_end_l1"=w97:i32)  [unwired: 11 in]
  n206 = call "BRig_dataCurrent_L_ENL_T_start_l2.vi"() -> ("output_L_T_ENL1_start_l2"=w95:i32)  [unwired: 11 in]
  n207 = call "BRig_dataCurrent_L_ENL_T_end_l2.vi"() -> ("output_L_ENL_T_end_l2"=w93:i32)  [unwired: 11 in]
  n208 = call "BRig_dataCurrent_L_ENL2_T_start_l1.vi"() -> ("output_L_ENL2_T_start_l1"=w36:i32)  [unwired: 11 in]
  n209 = call "BRig_dataCurrent_L_ENL2_T_end_l1.vi"() -> ("output_L_ENL2_T_end_l1"=w34:i32)  [unwired: 11 in]
  n210 = call "BRig_dataCurrent_L_ENL2_T_start_l2.vi"() -> ("output_L_T_ENL2_start_l2"=w32:i32)  [unwired: 11 in]
  n211 = call "BRig_dataCurrent_L_ENL2_T_end_l2.vi"() -> ("output_L_ENL2_T_end_l2"=w30:i32)  [unwired: 11 in]
  n212 = Replace Array Subset(array="input_dataCurrent", new element #1=w98, index #1=w99, new element #2=w96, index #2=w97, new element #3=w94, index #3=w95, new element #4=w92, index #4=w93, new element #5=w35, index #5=w36, new element #6=w33, index #6=w34, new element #7=w31, index #7=w32, new element #8=w29, index #8=w30) -> (→"output_dataCurrent":u16[])
  n213 = call "BRig_dataTrial_L_ENL_event_I_l1.vi"() -> ("output_L_ENL_event_I_l1"=w114:i32)  [unwired: 11 in]
  n214 = call "BRig_dataTrial_L_ENL_trig_I_l1.vi"() -> ("output_L_ENL_trig_I_l1"=w111:i32)  [unwired: 11 in]
  n215 = call "BRig_dataTrial_L_ENL_event_I_l2.vi"() -> ("output_L_ENL_event_I_l2"=w110:i32)  [unwired: 11 in]
  n216 = call "BRig_dataTrial_L_ENL_trig_I_l2.vi"() -> ("output_L_ENL_trig_I_l2"=w109:i32)  [unwired: 11 in]
  n217 = call "BRig_dataTrial_L_ENL2_event_I_l1.vi"() -> ("output_L_ENL2_event_I_l1"=w64:i32)  [unwired: 11 in]
  n218 = call "BRig_dataTrial_L_ENL2_trig_I_l1.vi"() -> ("output_L_ENL2_trig_I_l1"=w63:i32)  [unwired: 11 in]
  n219 = call "BRig_dataTrial_L_ENL2_event_I_l2.vi"() -> ("output_L_ENL2_event_I_l2"=w62:i32)  [unwired: 11 in]
  n220 = call "BRig_dataTrial_L_ENL2_trig_I_l2.vi"() -> ("output_L_ENL2_trig_I_l2"=w60:i32)  [unwired: 11 in]
  n221 = call "BRig_arrTrig_L_ENL_event_l1.vi"() -> ("output_L_ENL_event_l1"=w122:i32)  [unwired: 11 in]
  n222 = call "BRig_arrTrig_L_ENL_laser_l1.vi"() -> ("output_L_ENL_laserTrig_l1"=w121:i32)  [unwired: 11 in]
  n223 = call "BRig_arrTrig_L_ENL_event_l2.vi"() -> ("output_L_ENL_event_l2"=w120:i32)  [unwired: 11 in]
  n224 = call "BRig_arrTrig_L_ENL_laser_l2.vi"() -> ("output_L_ENL_laserTrig_l2"=w119:i32)  [unwired: 11 in]
  n225 = call "BRig_arrTrig_L_ENL2_event_l1.vi"() -> ("output_L_ENL2_event_l1"=w72:i32)  [unwired: 11 in]
  n226 = call "BRig_arrTrig_L_ENL2_laser_l1.vi"() -> ("output_L_ENL2_laserTrig_l1"=w71:i32)  [unwired: 11 in]
  n227 = call "BRig_arrTrig_L_ENL2_event_l2.vi"() -> ("output_L_ENL2_event_l2"=w70:i32)  [unwired: 11 in]
  n228 = call "BRig_arrTrig_L_ENL2_laser_l2.vi"() -> ("output_L_ENL2_laserTrig_l2"=w69:i32)  [unwired: 11 in]
  n229 = Boolean To (0,1)(Boolean=w113) -> (0, 1=w118:i16)
  n230 = Boolean To (0,1)(Boolean=w107) -> (0, 1=w117:i16)
  n231 = Boolean To (0,1)(Boolean=w105) -> (0, 1=w115:i16)
  n232 = Boolean To (0,1)(Boolean=w103) -> (0, 1=w116:i16)
  n233 = Boolean To (0,1)(Boolean=w40) -> (0, 1=w68:i16)
  n234 = Boolean To (0,1)(Boolean=w39) -> (0, 1=w67:i16)
  n235 = Boolean To (0,1)(Boolean=w38) -> (0, 1=w65:i16)
  n236 = Boolean To (0,1)(Boolean=w37) -> (0, 1=w66:i16)
  n237 = Replace Array Subset(array="input_arrTrig", new element #1=w113, index #1=w122, new element #2=w107, index #2=w121, new element #3=w105, index #3=w120, new element #4=w103, index #4=w119, new element #5=w40, index #5=w72, new element #6=w39, index #6=w71, new element #7=w38, index #7=w70, new element #8=w37, index #8=w69) -> (→"output_arrTrig":bool[])
  n238 = To Unsigned Word Integer(number=w118) -> (unsigned 16bit integer=w112:u16)
  n239 = To Unsigned Word Integer(number=w117) -> (unsigned 16bit integer=w108:u16)
  n240 = To Unsigned Word Integer(number=w115) -> (unsigned 16bit integer=w106:u16)
  n241 = To Unsigned Word Integer(number=w116) -> (unsigned 16bit integer=w104:u16)
  n242 = To Unsigned Word Integer(number=w68) -> (unsigned 16bit integer=w59:u16)
  n243 = To Unsigned Word Integer(number=w67) -> (unsigned 16bit integer=w58:u16)
  n244 = To Unsigned Word Integer(number=w65) -> (unsigned 16bit integer=w57:u16)
  n245 = To Unsigned Word Integer(number=w66) -> (unsigned 16bit integer=w56:u16)
  n246 = Replace Array Subset(array="input_dataTrial", new element #1=w112, index (row) #1=w61, index (col) #1=w114, new element #2=w108, index (row) #2=w61, index (col) #2=w111, new element #3=w106, index (row) #3=w61, index (col) #3=w110, new element #4=w104, index (row) #4=w61, index (col) #4=w109, new element #5=w59, index (row) #5=w61, index (col) #5=w64, new element #6=w58, index (row) #6=w61, index (col) #6=w63, new element #7=w57, index (row) #7=w61, index (col) #7=w62, new element #8=w56, index (row) #8=w61, index (col) #8=w60) -> (→"output_dataTrial":u16[][])
